vi "Special Write.vi"(8 "error in (no error)":errorcluster, 9 "Send String":string, 11 "VISA resource name":refnum<visa-resource-name>) -> (0 "error out":errorcluster, 1 "Parsed Response String":string, 2 "Status":u16(ring) items=["Ready", "Busy"], 3 "VISA resource name out":refnum<visa-resource-name>, 4 "Unparsed Response String":string)   [LabVIEW 2021, in "Copy of Kloehn V6 Series.lvlib"]
doc: "Writes the string to the instrument and receives the reply with the parsed response. The parsed response comes in handy for reads or queries for the instrument."
uses:
  Copy of Kloehn V6 Series.lvlib
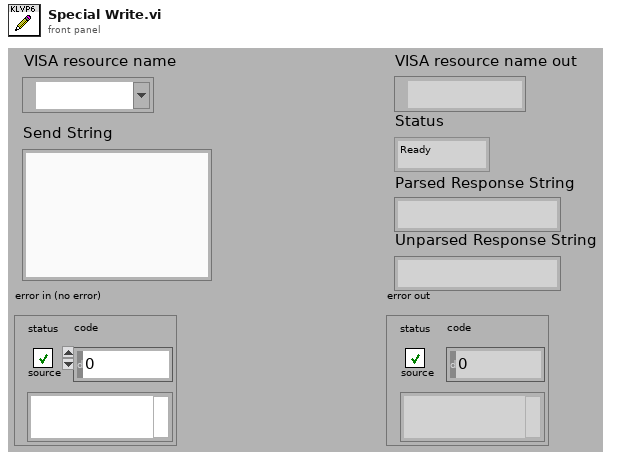
[diagram p1: front panel]
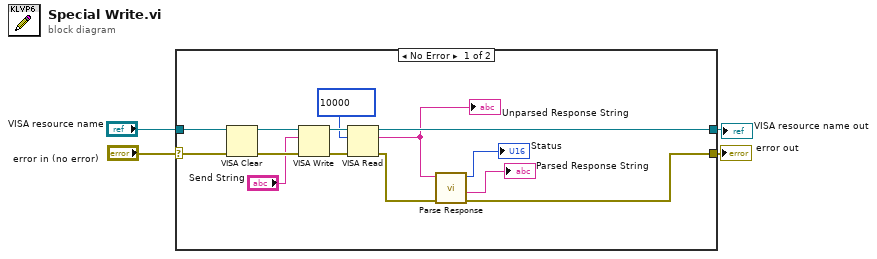
[diagram p0: block diagram]
diagram:
  n1 = case shown="No Error" "error in (no error)" {
    selector: "error in (no error)" -> [w15 w20]
    tunnel: "VISA resource name" -> [w14 w19]
    tunnel: [w8 w20] -> w3
    tunnel: [w11 w19] -> w1
    frame No Error {
      n2 = VISA Clear(VISA resource name=w14, error in (no error)=w15) -> (VISA resource name out=w12:refnum<visa-resource-name>, error out=w13:errorcluster)
      n3 = VISA Write(VISA resource name=w12, write buffer="Send String", error in (no error)=w13) -> (VISA resource name out=w17:refnum<visa-resource-name>, error out=w18:errorcluster)  [unwired: 1 out]
      n4 = VISA Read(VISA resource name=w17, byte count=u32 10000, error in (no error)=w18) -> (VISA resource name out=w11:refnum<visa-resource-name>, read buffer=w10:string, error out=w9:errorcluster)  [unwired: 1 out]
      "Unparsed Response String" <- w10
      n5 = call "Parse Response.vi"("error in (no error)"=w9, "Send String"=w10) -> ("error out"=w8:errorcluster, "Response String"=→"Parsed Response String":string, "Status"=→"Status":u16)  [unwired: 7 in]
    }
    frame Error {
    }
  }
  "error out" <- w3
  "VISA resource name out" <- w1
